vi "Execute.vi"(6 "Index [-1]":i32=-1, 7 "Composite Object":refnum<class "CConfig Object.lvclass">, 8 "error in (no error)":errorcluster, 9 "Results":string[][](array[string]), 11 "Config Query in":refnum<class "Search Replace Query.lvclass">) -> (0 "error out":errorcluster, 1 "Results":string[][](array[string]), 2 "Result":bool, 3 "Config Query out":refnum<class "Search Replace Query.lvclass">, 4 "Index":i32, 5 "Composite Object":refnum<class "CConfig Object.lvclass">)   [LabVIEW 2013, in "Search Replace Query.lvclass"]
doc: "Copyright 2018, Carya Automatisering, Wiebe Walstra."
uses:
  Search Replace Query.lvclass
  CConfig Object.lvclass
  Search Replace Query.lvclass/Search Replace Query.ctl
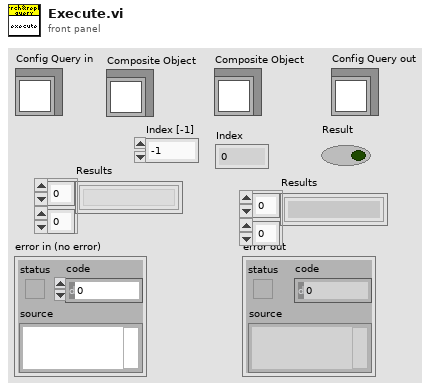
[diagram p1: front panel]
types:
  T1 = typedef "CConfig Object.lvclass/Data.ctl" = enum16{"pre", "name", "middle", "value", "post", "newline", "persistant", "tagged", "type"}
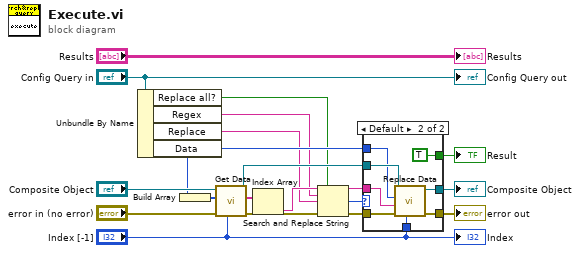
[diagram p0: block diagram]
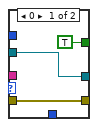
[diagram p2: hidden frame]
diagram:
  n1 = Unbundle By Name("Config Query in") -> ("Replace all?"=w1:bool, "Regex"=w6:string, "Replace"=w5:string, "Data"=w12:T1)
  n2 = Build Array(w12) -> (w16:T1[])
  n3 = call-dynamic "Get Data.vi"("Index in"="Index [-1]", "error in (no error)"="error in (no error)", "Data"=w16, "Composite Object in"="Composite Object") -> ("error out"=w9:errorcluster, "Data"=w10:string[], "Composite Object out"=w14:refnum<class "CConfig Object.lvclass">)  [unwired: 5 in]
  n4 = Index Array(array=w10) -> (element=w7:string)  [unwired: 1 in]
  n5 = Search and Replace String(replace all?=w1, input string=w7, search string=w6, replace string=w5, error in=w9) -> (result string=w4:string, number of replacements=w3:i32, error out=w8:errorcluster)  [unwired: 3 in, 1 out]
  n6 = case shown="Default" w3 {
    tunnel: [w22 w31] -> w15
    tunnel: w14 -> [w23 w30]
    tunnel: [w23 w29] -> w13
    tunnel: w12 -> [_ w28]
    tunnel: "Index [-1]" -> [_ w27]
    tunnel: w8 -> [w22 w26]
    tunnel: w4 -> [_ w25]
    tunnel: [TRUE ("Result") TRUE ("Result")] -> w2
    frame 0 {
    }
    frame Default {
      n7 = call-dynamic "Replace Data.vi"("Index in"=w27, "error in (no error)"=w26, "Value"=w25, "Data"=w28, "Composite Object in"=w30) -> ("error out"=w31:errorcluster, "Composite Object out"=w29:refnum<class "CConfig Object.lvclass">)  [unwired: 5 in]
    }
  }
  "error out" <- w15
  "Composite Object" <- w13
  "Result" <- w2
  "Config Query out" <- "Config Query in"
  "Index" <- "Index [-1]"
  "Results" <- "Results"
